vi "Get Scanner (basic).vi"(8 "error in (no error)":errorcluster, 11 "Pulse Generator in":refnum<class "Pulse Generator.lvclass">) -> (0 "error out":errorcluster, 2 "Pulse Gen Basic Scanner out":refnum<class "Scanner.lvclass">)   [LabVIEW 2017, in "Pulse Generator.lvclass"]
doc: "(Dynamic) Returns the default Scanner object that scans over this Scannable. (Note that a Scannable may have multiple Scanners associated with it.) A Scanner is an analogue to an Iterator class in other languages."
uses:
  Pulse Generator.lvclass
  Scanners/Scanner/Scanner.lvclass
  Scanners/Pulse Gen Basic Scan/Pulse Gen Basic Scan.lvclass
  C:/LabVIEW-programs/Scanners/Scanner/Scanner.lvclass
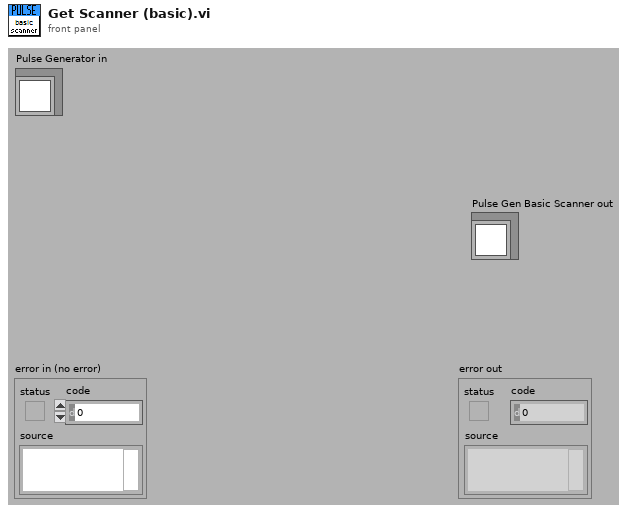
[diagram p1: front panel]
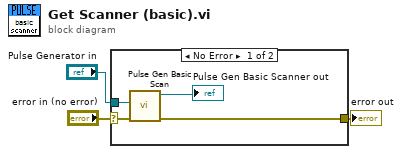
[diagram p0: block diagram]
diagram:
  n1 = case shown="No Error" "error in (no error)" {
    selector: "error in (no error)" -> [w6 w8]
    tunnel: [w7 w8] -> w2
    tunnel: "Pulse Generator in" -> [w5 _]
    frame No Error {
      n2 = call "Pulse Gen Basic Scan.vi"("error in (no error)"=w6, "Pulse Generator.lvclass"=w5) -> ("error out"=w7:errorcluster, "Pulse Gen Basic Scan out"=→"Pulse Gen Basic Scanner out":refnum<class "Pulse Gen Basic Scan.lvclass">)  [unwired: 8 in]
    }
    frame Error {
    }
  }
  "error out" <- w2
